vi "CaseExample.vi"() -> ()   [LabVIEW 2020]
doc: "Example of case structure with most common data types which can be used as selector . Comments in polish language."
panel:
  out "Information out 2":string
  out "Information out":string
  in  "Enum":T1(ring)
  in  "Numeric":u8
  in  "String":string
  in  "Boolean":bool
  out "Error Out":errorcluster
  in  "Error In":errorcluster
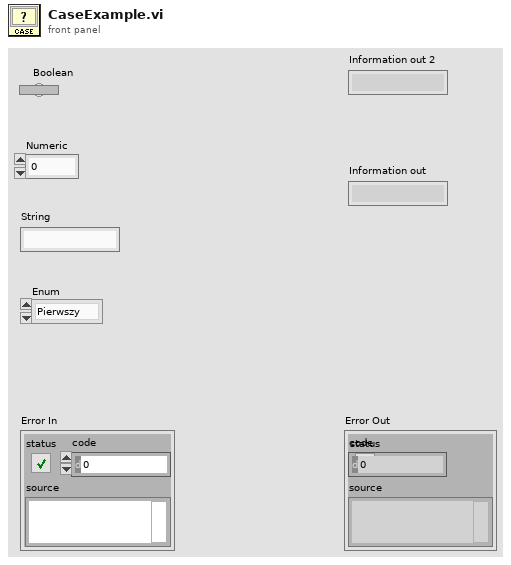
[diagram p1: front panel]
types:
  T1 = enum16{"Pierwszy ", "Drugi", "Trzeci", "Czwarte"}
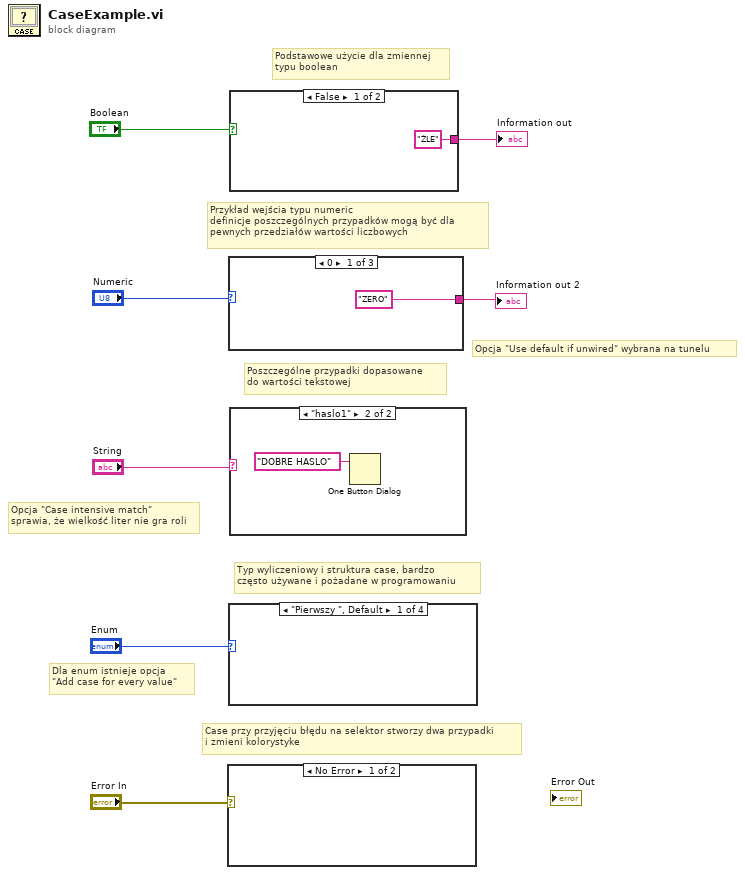
[diagram p0: block diagram]
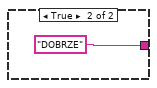
[diagram p2: hidden frame]
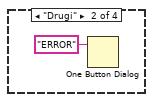
[diagram p6: hidden frame]
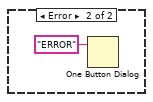
[diagram p9: hidden frame]
diagram:
  # "Case przy przyjęciu błędu na selektor stworzy dwa przypadki\ni zmieni kolorystyke"
  # "Dla enum istnieje opcja \n\"Add case for every value\""
  # "Typ wyliczeniowy i struktura case, bardzo\nczęsto używane i pożadane w programowaniu"
  # "Poszczególne przypadki dopasowane \ndo wartości tekstowej"
  # "Opcja \"Case intensive match\"\nsprawia, że wielkość liter nie gra roli"
  # "Opcja \"Use default if unwired\" wybrana na tunelu"
  # "Przykład wejścia typu numeric\ndefinicje poszczególnych przypadków mogą być dla \npewnych przedziałów wartości liczbowych"
  # "Podstawowe użycie dla zmiennej\ntypu boolean"
  n1 = case shown="No Error" "Error In" {
    frame No Error {
    }
    frame Error {
      n2 = One Button Dialog(message="ERROR") -> ()  [unwired: 1 in, 1 out]
    }
  }
  n3 = case shown="0" "Numeric" {
    tunnel: ["ZERO" ("Information out 2") _ _] -> w1
    frame 0 {
    }
    frame 1..5 {
    }
    frame 7, Default {
    }
  }
  "Information out 2" <- w1
  n4 = case shown="\"Pierwszy \", Default" "Enum" {
    frame "Pierwszy ", Default {
    }
    frame "Drugi" {
      n5 = One Button Dialog(message="ERROR") -> ()  [unwired: 1 in, 1 out]
    }
    frame "Trzeci" {
    }
    frame "Czwarte" {
    }
  }
  n6 = case shown="False" "Boolean" {
    tunnel: ["ŹLE" "DOBRZE"] -> w2
    frame False {
    }
    frame True {
    }
  }
  "Information out" <- w2
  n7 = case shown="\"haslo1\"" "String" {
    frame Default {
    }
    frame "haslo1" {
      n8 = One Button Dialog(message="DOBRE HASLO") -> ()  [unwired: 1 in, 1 out]
    }
  }
